vi "Parse Raw Data.vi"(8 "error in":errorcluster, 11 "Raw Data":u8[](array[numeric]) format="%.0x") -> (1 "Board Out":T1, 3 "Modules Out":T1[](array[typedef]))   [LabVIEW 2018, in "Control Box.lvlib" / "Control Box.lvclass"]
uses:
  Control Box.lvclass
  Custom Controls/Channel Status.ctl
  Control Box.lvlib
panel:
  out "error out":errorcluster
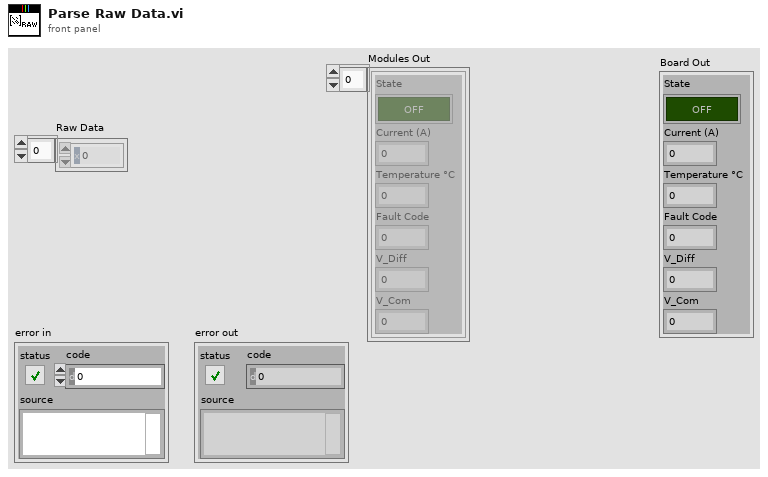
[diagram p1: front panel]
types:
  T1 = typedef "Control Box.lvlib/Channel Status.ctl" = cluster{"State":bool, "Current (A)":dbl, "Temperature °C":dbl, "Fault Code":u8, "V_Diff":dbl, "V_Com":dbl}
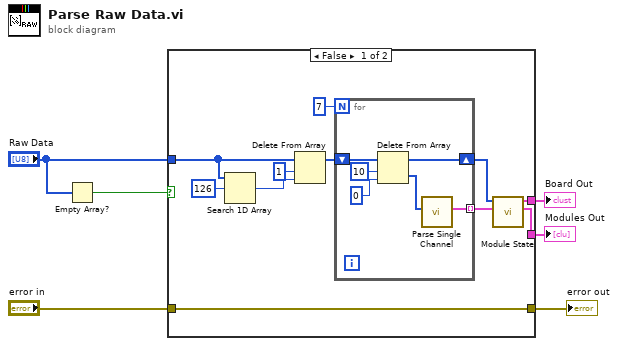
[diagram p0: block diagram]
diagram:
  n1 = Empty Array?(array="Raw Data") -> (empty?=w6:bool)
  n2 = case shown="False" w6 {
    tunnel: "Raw Data" -> [w16 _]
    tunnel: "error in" -> [w11 w24]
    tunnel: [w11 w24] -> w3
    tunnel: [w8 _] -> w1
    tunnel: [w7 _] -> w2
    frame False {
      n3 = Search 1D Array(1D array=w16, element=u8 126) -> (index of element=w15:i32)  [unwired: 1 in]
      n4 = Delete From Array(array=w16, length=1, index=w15) -> (array with subset deleted=w13:u8[])  [unwired: 1 out]
      n5 = for {
        N: 7 -> [_]
        shift-right: [w20] -> w9
        shift-left: w13 -> [w23]
        tunnel: [w18] -> w10 mode=indexing
        n6 = Delete From Array(array=w23, length=10, index=0) -> (deleted portion=w19:u8[], array with subset deleted=w20:u8[])
        n7 = call "Parse Single Channel.vi"("Raw Data"=w19) -> ("Channel"=w18:T1)  [unwired: 10 in]
      }
      n8 = call "Module State.vi"("Modules In"=w10, "Data In"=w9) -> ("Modules Out"=w7:T1[], "Board Out"=w8:T1)  [unwired: 8 in]
    }
    frame True {
    }
  }
  "error out" <- w3
  "Modules Out" <- w2
  "Board Out" <- w1
